vi "AC_6011_AD.vi"(2 "times":i32, 3 "ch":i32, 4 "idd(out)":u32, 5 "hDevice(in)":u32) -> (0 "hDevice(out)":u32, 1 "data":i32)   [LabVIEW 2015]
uses:
  acpci.dll
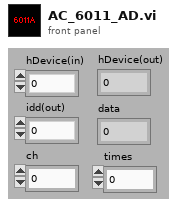
[diagram p1: front panel]
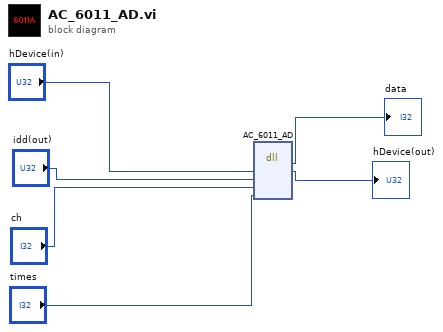
[diagram p0: block diagram]
diagram:
  n1 = dll-call lib="PTH2|abs F2.技术库labviewVI小程序:基于Labview的直流伺服电机位置控制系统设计\t源程序\tACPCI.DLL" fn="AC_6011_AD"("hDevice"="hDevice(in)", "idd"="idd(out)", "ch"="ch", "times"="times") -> (→"data":u32, "hDevice"=→"hDevice(out)":u32)  [unwired: 6 in, 2 out]
